vi "runTestScenario.vi"(8 "error in (no error)":errorcluster, 11 "ITestScenario in":refnum<class "NotImplementedTest.lvclass">) -> (0 "error out":errorcluster, 1 "Result":T1, 2 "TestExecution":T2, 3 "ITestScenario out":refnum<class "NotImplementedTest.lvclass">)   [LabVIEW 2015, in "NotImplementedTest.lvclass"]
uses:
  NotImplementedTest.lvclass
  Typedefs/TestExecution.ctl
  Typedefs/PassFailTest.ctl
  Typedefs/ILCBTTypedefs.lvlib
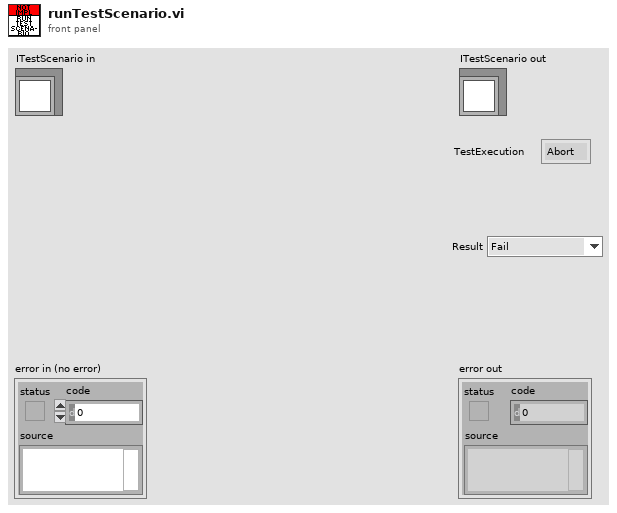
[diagram p1: front panel]
types:
  T1 = typedef "ILCBTTypedefs.lvlib/PassFailTest.ctl" = enum16{"Fail", "Pass", "NA"}
  T2 = typedef "ILCBTTypedefs.lvlib/TestExecution.ctl" = enum16{"Abort", "Continue"}
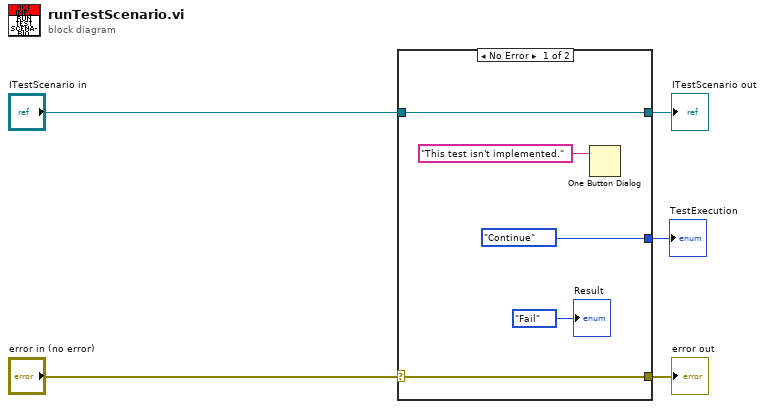
[diagram p0: block diagram]
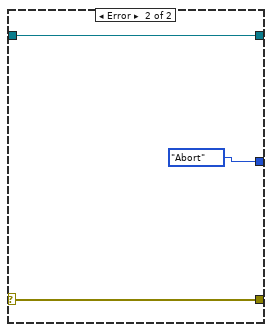
[diagram p2: hidden frame]
diagram:
  n1 = case shown="No Error" "error in (no error)" {
    selector: "error in (no error)" -> [w9 w13]
    tunnel: [w9 w13] -> w4
    tunnel: [w10 w12] -> w2
    tunnel: "ITestScenario in" -> [w10 w12]
    tunnel: [TestExecution."Continue" ("TestExecution") TestExecution."Abort" ("TestExecution")] -> w1
    frame No Error {
      n2 = One Button Dialog(message="This test isn't implemented.") -> ()  [unwired: 1 in, 1 out]
      "Result" <- PassFailTest."Fail" ("Result")
    }
    frame Error {
    }
  }
  "error out" <- w4
  "ITestScenario out" <- w2
  "TestExecution" <- w1
